vi "Target Shift Prosthesis Angle to Ankle Angle.vi"(11 "Prosthesis Angle (deg)":dbl) -> (3 "Ankle Angle (deg)":dbl)   [LabVIEW 2018, in "COBRA Measurement and Filtering Library.lvlib"]
uses:
  COBRA Measurement and Filtering Library.lvlib
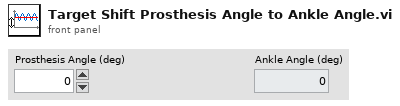
[diagram p1: front panel]
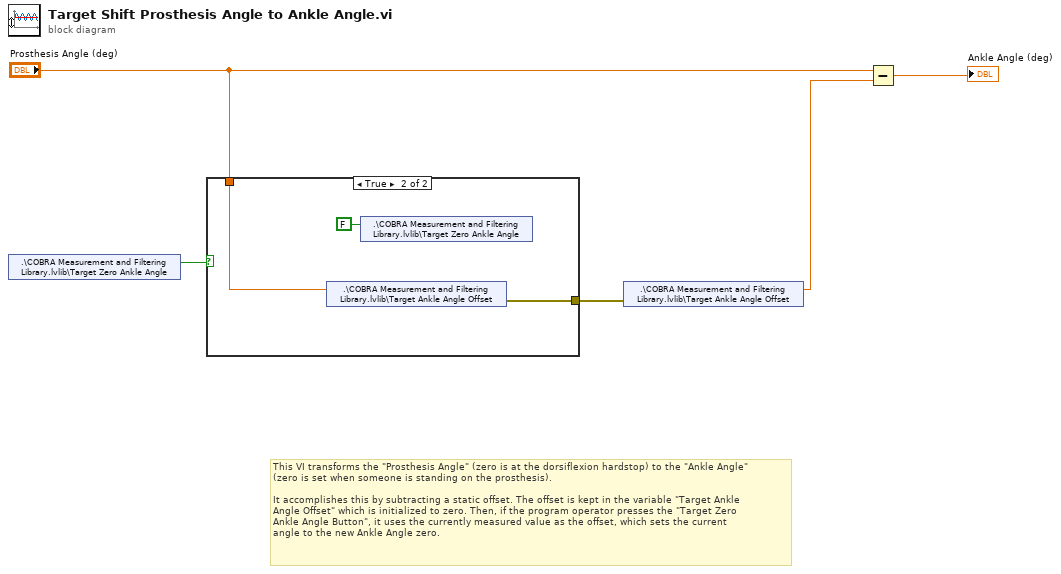
[diagram p0: block diagram]
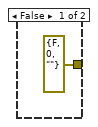
[diagram p2: hidden frame]
diagram:
  # "This VI transforms the \"Prosthesis Angle\" (zero is at the dorsiflexion hardstop) to the \"Ankle Angle\"\n(zero is set when someone is standing on the prosthesis).\n\nIt accomplishes this by subtracting a static offset. The offset is kept in the variable \"Target Ankle\nAngle Offset\" which is initialized to zero. Then, if the program operator presses the \"Target Zero\nAnkle Angle Button\", it uses the currently measured value as the offset, which sets the current\nangle to the new Ankle Angle zero."
  n1 = shared-variable ".\\COBRA Measurement and Filtering Library.lvlib\\Target Zero Ankle Angle"() -> (w4:bool)  [unwired: 1 in, 1 out]
  n2 = case shown="True" w4 {
    tunnel: "Prosthesis Angle (deg)" -> [_ w8]
    tunnel: [errorcluster {"status"=FALSE, "code"=0, "source"=""} ("error IO") w7] -> w2
    frame False {
    }
    frame True {
      n3 = shared-variable ".\\COBRA Measurement and Filtering Library.lvlib\\Target Ankle Angle Offset"(w8) -> (error out=w7:errorcluster)  [unwired: 1 in]
      n4 = shared-variable ".\\COBRA Measurement and Filtering Library.lvlib\\Target Zero Ankle Angle"(FALSE ("Target Zero Ankle Angle")) -> ()  [unwired: 1 in, 1 out]
    }
  }
  n5 = shared-variable ".\\COBRA Measurement and Filtering Library.lvlib\\Target Ankle Angle Offset"(error in=w2) -> (w1:dbl)  [unwired: 1 out]
  n6 = Subtract(x="Prosthesis Angle (deg)", y=w1) -> (x-y=→"Ankle Angle (deg)":dbl)
